vi "sendValue.vi"(8 "error in (no error)":errorcluster, 10 "data":variant, 11 "openShutter in":refnum<class "openShutter.lvclass">) -> (0 "error out":errorcluster, 2 "function return":i32, 3 "openShutter out":refnum<class "openShutter.lvclass">)   [LabVIEW 2016, in "SALLV_AtDome_Messaging.lvlib" / "openShutter.lvclass"]
uses:
  openShutter.lvclass
  ts_sallv_AtDome/DataTypes/command_closeShutter.ctl
  ts_sallv_AtDome/SALLV_AtDome.lvlib
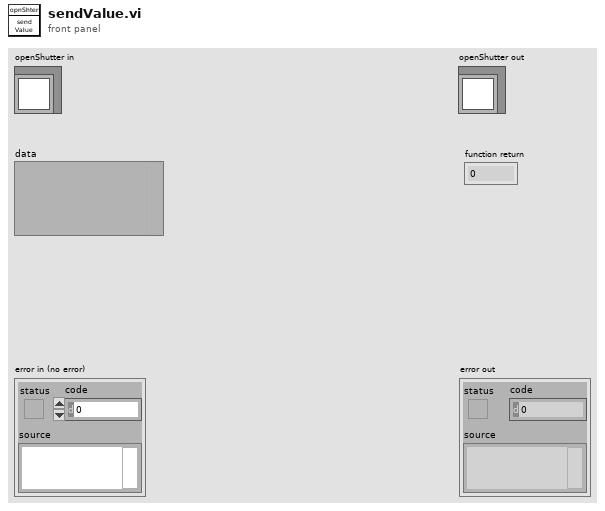
[diagram p1: front panel]
types:
  T1 = typedef "SALLV_AtDome.lvlib/command_closeShutter.ctl" = cluster{"close":bool}
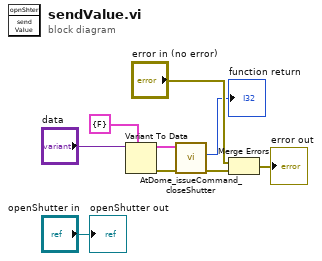
[diagram p0: block diagram]
diagram:
  n1 = Variant To Data(type=T1 {"close"=FALSE} ("data"), Variant="data") -> (data=w3:T1, error out=w4:errorcluster)  [unwired: 1 in]
  n2 = call "AtDome_issueCommand_closeShutter.vi"("error in (no error)"=w4, "command_closeShutter_Ctl"=w3) -> ("error out"=w5:errorcluster, "function return"=→"function return":i32)  [unwired: 7 in, 1 out]
  n3 = Merge Errors("error in (no error)", w5) -> (→"error out":errorcluster)
  "openShutter out" <- "openShutter in"
